vi "Abort VI On Stop Event.vi"(0 "VI Reference":refnum<vi>) -> ()   [LabVIEW 2013]
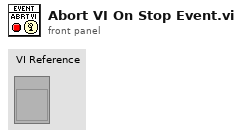
[diagram p1: front panel]
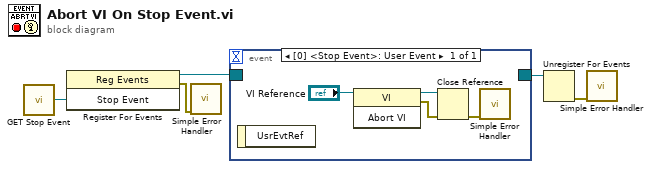
[diagram p0: block diagram]
diagram:
  n1 = call "GET Stop Event.vi"() -> ("Stop Event"=w5:refnum<user-event>)
  n2 = register-events(w5) -> (reference out=w4:refnum<event-registration>, error out=w3:errorcluster)  [unwired: 2 in]
  n3 = call <vilib>:"Simple Error Handler.vi"("error in (no error)"=w3) -> ()  [unwired: 4 in, 5 out]
  n4 = event shown="[0] <Stop Event>: User Event" {
    selector: w4 -> [_]
    dyn-events: [_] -> w2
    timeout: _ -> [_]
    event User Event {
      n5 = event-data() -> ()  [unwired: 1 in, 1 out]
      n6 = invoke class="VI" method="Abort VI"(reference="VI Reference") -> (reference out=w7:refnum<vi>, error out=w8:errorcluster)  [unwired: 2 in, 1 out]
      n7 = Close Reference(reference=w7, error in (no error)=w8) -> (error out=w9:errorcluster)
      n8 = call <vilib>:"Simple Error Handler.vi"("error in (no error)"=w9) -> ()  [unwired: 4 in, 5 out]
    }
  }
  n9 = Unregister For Events(event registration refnum=w2) -> (error out=w1:errorcluster)  [unwired: 1 in]
  n10 = call <vilib>:"Simple Error Handler.vi"("error in (no error)"=w1) -> ()  [unwired: 4 in, 5 out]
